vi "Temp Tester for CT.vi"() -> ()   [LabVIEW 2016]
uses:
  type defs/ERD Read List All.ctl
  Q:/Common/DLLs/GEA3/GeaCommunication.dll
  Common/DLLs/GEA3/GeaCommunication.dll
  Common/LabVIEW GEA2 Toolkit/LabVIEW_GEA2_Toolkit.lvlibp/type defs/ERD Read Data Out.ctl
  Common/LabVIEW GEA2 Toolkit/LabVIEW_GEA2_Toolkit.lvlibp/type defs/Source_Destination.ctl
  <vilib>/DAQmx/write.llb/DAQmx Write (Analog 1D DBL NChan 1Samp).vi
  <vilib>/DAQmx/create/channels.llb/DAQmx Create Channel (AO-Voltage-Basic).vi
  <vilib>/DAQmx/miscellaneous.llb/DAQmx Fill In Error Info.vi
  <vilib>/Utility/file.llb/Write Delimited Spreadsheet (DBL).vi
  Common/LabVIEW GEA2 Toolkit/LabVIEW_GEA2_Toolkit.lvlibp
panel:
  out "Array 2":dbl[](array[numeric])
  out "Array":string[](array[string])
  out "ERD Output":T1 {"ERD Number" format="%.0x"}
  in  "Varry Inlet":bool
  in  "Vary Outlet?":bool
  in  "GEA2 Reference In":refnum<k24>
  out "GEA2 Reference Out":refnum<k24>
  out "Error Out":errorcluster
  in  "Delay":u32=2000
  out "error out":errorcluster
  in  "File Path Control":path
  in  "Filtered Moisture":dbl
  in  "ERD Read List ALL":T2=[{"Boolean"=TRUE, "ERD Number"=62475, "ERD Name"="Machine State", "Data Type"=enum."uint8_t"}, {"Boolean"=TRUE, "ERD Number"=62465, "ERD Name"="Relay Status", "Data Type"=enum."string"}, {"Boolean"=TRUE, "ERD Number"=62467, "ERD Name"="Door Switch State", "Data Type"=enum."string"}, {"Boolean"=TRUE, "ERD Number"=62468, "ERD Name"="Door Latch State", "Data Type"=enum."string"}, {"Boolean"=TRUE, "ERD Number"=62469, "ERD Name"="Inlet Thermistor", "Data Type"=enum."int16_t"}, {"Boolean"=TRUE, "ERD Number"=62470, "ERD Name"="Outlet Thermistor", "Data Type"=enum."int16_t"}, {"Boolean"=TRUE, "ERD Number"=62471, "ERD Name"="Filtered Moisture", "Data Type"=enum."int16_t"}, {"Boolean"=TRUE, "ERD Number"=62476, "ERD Name"="Control Lock State", "Data Type"=enum."string"}, {"Boolean"=TRUE, "ERD Number"=62491, "ERD Name"="Signal Volume", "Data Type"=enum."string"}, {"Boolean"=TRUE, "ERD Number"=62478, "ERD Name"="Drum Light", "Data Type"=enum."string"}, {"Boolean"=TRUE, "ERD Number"=62486, "ERD Name"="Delay Time", "Data Type"=enum."string"}, {"Boolean"=TRUE, "ERD Number"=62507, "ERD Name"="Ext. Tumble", "Data Type"=enum."string"}, {"Boolean"=TRUE, "ERD Number"=62487, "ERD Name"="Cycle Time", "Data Type"=enum."uint32_t"}, {"Boolean"=TRUE, "ERD Number"=62488, "ERD Name"="Sub-Cycle", "Data Type"=enum."uint8_t"}, {"Boolean"=TRUE, "ERD Number"=62497, "ERD Name"="Temp Level", "Data Type"=enum."string"}, {"Boolean"=TRUE, "ERD Number"=62499, "ERD Name"="Dryness Level", "Data Type"=enum."string"}, {"Boolean"=TRUE, "ERD Number"=62501, "ERD Name"="eDry", "Data Type"=enum."string"}, {"Boolean"=TRUE, "ERD Number"=62505, "ERD Name"="Time Level", "Data Type"=enum."string"}, {"Boolean"=TRUE, "ERD Number"=62509, "ERD Name"="Damp Alert", "Data Type"=enum."string"}, {"Boolean"=TRUE, "ERD Number"=62511, "ERD Name"="Detangle", "Data Type"=enum."string"}, {"Boolean"=TRUE, "ERD Number"=62520, "ERD Name"="MyCycle", "Data Type"=enum."string"}, {"Boolean"=TRUE, "ERD Number"=62721, "ERD Name"="Cycle Engine State", "Data Type"=enum."string"}, {"Boolean"=TRUE, "ERD Number"=62724, "ERD Name"="Cycle Selected", "Data Type"=enum."string"}] {"ERD Number" format="%.0x"}
  in  "Inlet Temp Voltage":dbl
  in  "Outlet Temp Voltage":dbl
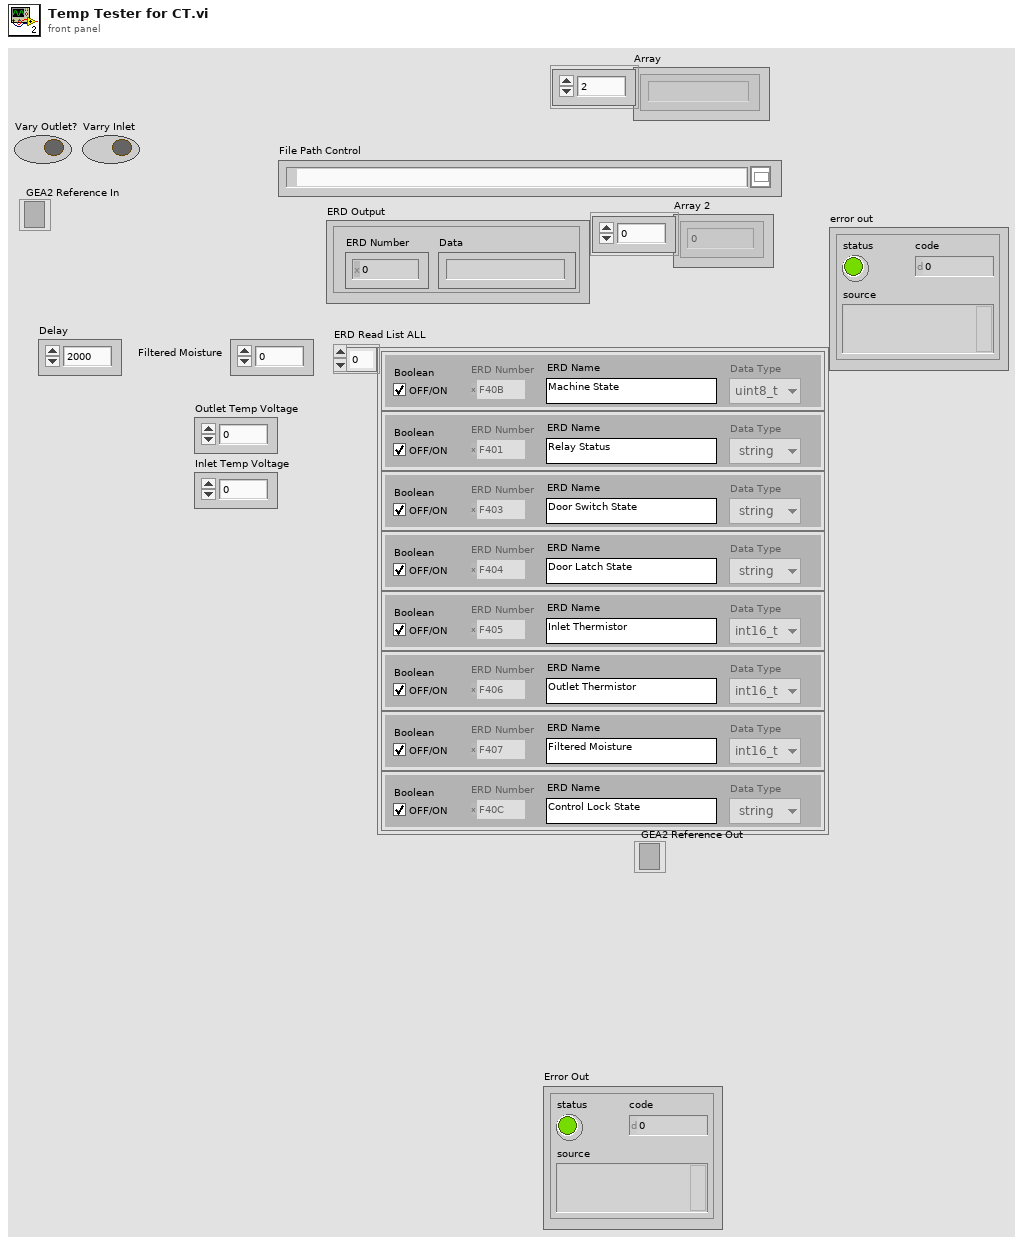
[diagram p1: front panel]
types:
  T1 = typedef "LabVIEW_GEA2_Toolkit.lvlibp/ERD Read Data Out.ctl" = cluster{"ERD Number":u16, "Data":string}
  T2 = typedef "ERD Read List All.ctl" = cluster{"Boolean":bool, "ERD Number":u16, "ERD Name":string, "Data Type":enum16{"string", "boolean", "uint8_t", "uint16_t", "uint32_t", "uint64_t", "int8_t", "int16_t", "int32_t", "int64_t"}}[]
  T3 = enum16{"open", "replace", "create", "open or create", "replace or create", "replace or create with confirmation"}
  T4 = enum16{"Init DAQ", "Build ERD List", "Set Voltage", "Read ERDs ", "Log Data", "Shut Down"}
  T5 = typedef "LabVIEW_GEA2_Toolkit.lvlibp/Source_Destination.ctl" = cluster{"Source":u8, "Destination":u8}
  T6 = typedef "LabVIEW_GEA2_Toolkit.lvlibp/ERD Read Data In.ctl" = cluster{"ERD Number":u16, "Data Type":T7}
  T7 = typedef "LabVIEW_GEA2_Toolkit.lvlibp/Data Type.ctl" = enum16{"string", "boolean", "uint8_t", "uint16_t", "uint32_t", "uint64_t", "int8_t", "int16_t", "int32_t", "int64_t"}
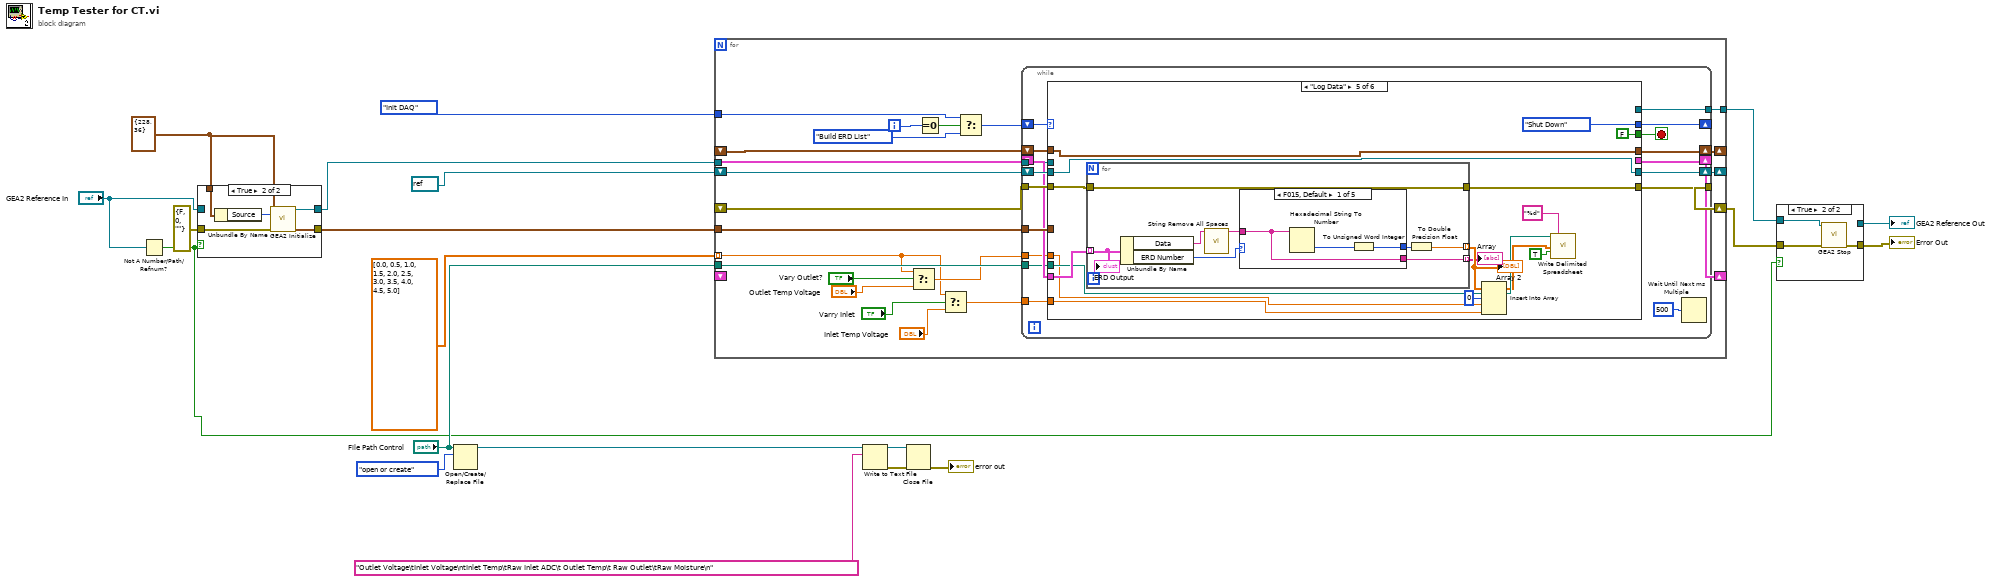
[diagram p0: block diagram]
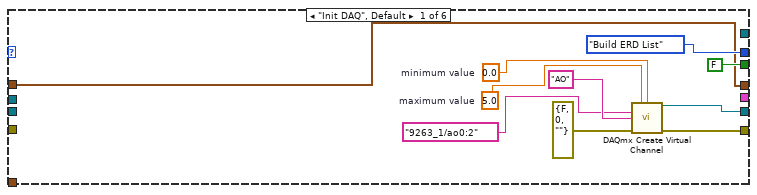
[diagram p4: hidden frame]
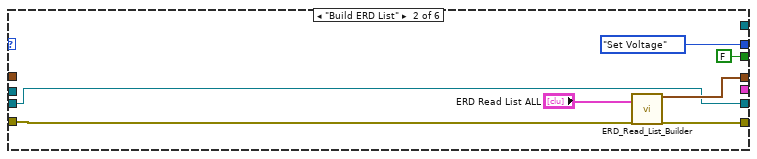
[diagram p5: hidden frame]
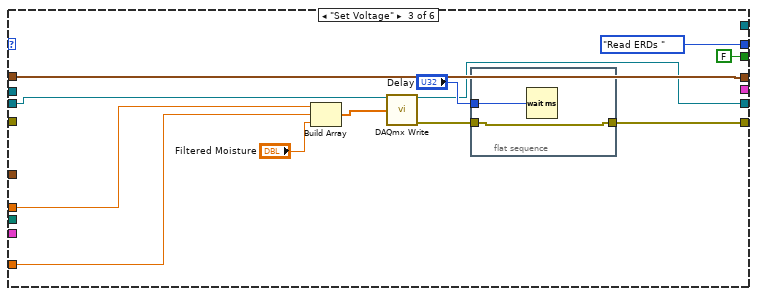
[diagram p6: hidden frame]
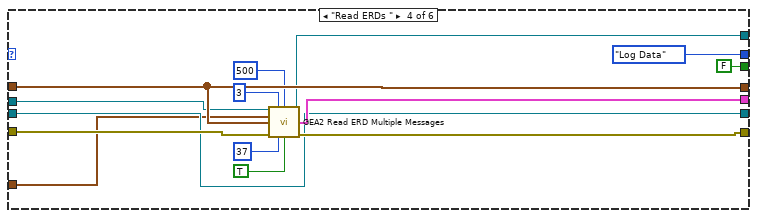
[diagram p7: hidden frame]
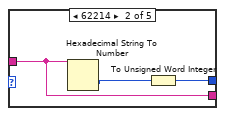
[diagram p8: hidden frame]
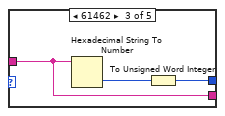
[diagram p9: hidden frame]
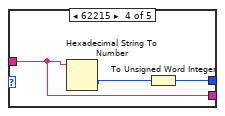
[diagram p10: hidden frame]
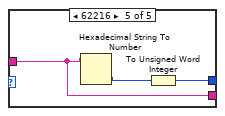
[diagram p11: hidden frame]
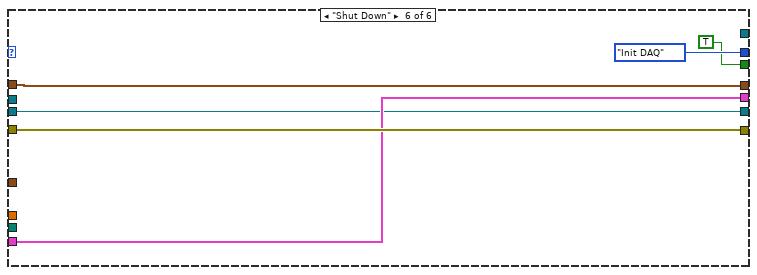
[diagram p12: hidden frame]
diagram:
  w8 = T5 {"Source"=228, "Destination"=36} ("GEA Inputs")
  n1 = Not A Number/Path/Refnum?(number/path/refnum="GEA2 Reference In") -> (NaN/Path/Refnum?=w4:bool)
  n2 = case shown="True" w4 {
    tunnel: errorcluster {"status"=FALSE, "code"=0, "source"=""} ("Error In") -> [w20 w26]
    tunnel: [w20 w25] -> _
    tunnel: "GEA2 Reference In" -> [w21 _]
    tunnel: [w21 w24] -> w9
    tunnel: w8 -> [_ w22]
    frame False {
    }
    frame True {
      n3 = Unbundle By Name(w22) -> ("Source"=w23:u8)
      n4 = call "GEA2 Initialize.vi"("Source Address"=w23, "error in"=w26) -> ("GEA2 Reference Out"=w24:refnum<k24>, "error out"=w25:errorcluster)  [unwired: 11 in, 1 out]
    }
  }
  n5 = Open/Create/Replace File(file path (use dialog)="File Path Control", operation (0:open)=T3."open or create") -> (refnum out=w15:refnum<file>)  [unwired: 4 in, 2 out]
  n6 = for {
    tunnel: w8 -> [w37]
    shift-right: [w38] -> _
    shift-left: refnum<k21> refnum ("task out") -> [w50]
    shift-right: [w49] -> w5
    shift-left: _ -> [w36]
    shift-right: [w48] -> _
    shift-left: _ -> [w47]
    shift-right: [w46] -> _
    shift-left: _ -> [w45]
    tunnel: dbl[] [0.0, 0.5, 1.0, 1.5, 2.0, 2.5, 3.0, 3.5, 4.0, 4.5, 5.0] -> [w32] mode=indexing
    tunnel: "File Path Control" -> [w44]
    tunnel: T4."Init DAQ" -> [w40]
    tunnel: w9 -> [w35]
    tunnel: [w34] -> w2
    i -> [w43]
    n7 = Select(t=w32, s="Vary Outlet?", f="Outlet Temp Voltage") -> (s? t:f=w33:dbl)
    n8 = Equal To 0?(x=w43) -> (x = 0?=w42:bool)
    n9 = Select(t=w32, s="Varry Inlet", f="Inlet Temp Voltage") -> (s? t:f=w31:dbl)
    n10 = Select(t=w40, s=w42, f=T4."Build ERD List") -> (s? t:f=w39:T4)
    n11 = while {
      tunnel: w37 -> [w65]
      tunnel: [w64] -> w49
      tunnel: w36 -> [w63]
      tunnel: w33 -> [w58]
      shift-right: [w67] -> _
      shift-left: w39 -> [w68]
      tunnel: w44 -> [w56]
      shift-right: [w55] -> w38
      shift-left: w50 -> [w66]
      tunnel: w35 -> [w53]
      shift-right: [w60] -> w46
      shift-left: w45 -> [w59]
      tunnel: [w52] -> w34
      shift-right: [w62] -> w48
      shift-left: w47 -> [w61]
      tunnel: w31 -> [w51]
      stop <- w57 stop-if-true
      n12 = case shown="\"Log Data\"" w68 {
        tunnel: [w75 w84 w91 w113 w124 w158] -> w64
        tunnel: [T4."Build ERD List" T4."Set Voltage" T4."Read ERDs " T4."Log Data" T4."Shut Down" T4."Init DAQ"] -> w67
        tunnel: [w72 w81 w89 w108 w129 w156] -> w55
        tunnel: w66 -> [_ w81 w88 w108 w129 w156]
        tunnel: w65 -> [_ _ _ w103 _ _]
        tunnel: w63 -> [_ w80 _ w112 w125 w158]
        tunnel: [w69 w82 w94 w109 w128 w155] -> w62
        tunnel: w61 -> [w69 _ w94 w109 w128 w155]
        tunnel: [_ _ _ w111 _ w157] -> w60
        tunnel: w59 -> [_ _ _ _ w126 w157]
        tunnel: w58 -> [_ _ w93 _ w118 _]
        tunnel: [FALSE FALSE FALSE FALSE FALSE TRUE] -> w57
        tunnel: w56 -> [_ _ _ _ w122 _]
        tunnel: w53 -> [_ _ _ w101 _ _]
        tunnel: [_ _ _ w100 _ _] -> w52
        tunnel: w51 -> [_ _ w86 _ w119 _]
        frame "Init DAQ", Default {
          w77 = 0.0  # minimum value
          w76 = 5.0  # maximum value
          n13 = call-poly <vilib>:"DAQmx Create Virtual Channel.vi"("maximum value"=w76, "minimum value"=w77, "physical channels"=tag "9263_1/ao0:2", "name to assign"="AO", "error in"=errorcluster {"status"=FALSE, "code"=0, "source"=""}) -> ("task out"=w72:refnum<k21>, "error out"=w75:errorcluster)  [unwired: 9 in]
        }
        frame "Build ERD List" {
          n14 = call "ERD_Read_List_Builder.vi"("ERD Read List"="ERD Read List ALL", "Error In"=w80) -> ("Read ERD List"=w82:T6[], "Error Out"=w84:errorcluster)  [unwired: 15 in, 1 out]
        }
        frame "Set Voltage" {
          n15 = Build Array(w93, w86, "Filtered Moisture") -> (w97:dbl[])
          n16 = call-poly <vilib>:"DAQmx Write.vi"("task/channels in"=w88, "data"=w97) -> ("task out"=w89:refnum<k21>, "error out"=w92:errorcluster)  [unwired: 11 in, 1 out]
          n17 = flat-sequence {
            tunnel: w92 -> [w99]
            tunnel: [w99] -> w91
            tunnel: "Delay" -> [w98]
            frame #0 {
              n18 = Wait (ms)(milliseconds to wait=w98) -> ()  [unwired: 1 out]
            }
          }
        }
        frame "Read ERDs " {
          n19 = call "GEA2 Read ERD Multiple Messages.vi"("GEA2 Reference In"=w101, "Retry Count"=3, "Read Timeout (ms)"=u32 500, "GEA Inputs"=w103, "Read ERD List"=w109, "Error In"=w112, "#ERDs per message"=37, "Verify ERD Response?"=TRUE) -> ("GEA2 Reference Out"=w100:refnum<k24>, "ERD Data Out"=w111:T1[], "Error Out"=w113:errorcluster)  [unwired: 4 in, 1 out]
        }
        frame "Log Data" {
          n20 = for {
            tunnel: w126 -> [w137] mode=indexing
            tunnel: w125 -> [w135]
            tunnel: [w135] -> w124
            tunnel: [w131] -> w120 mode=indexing
            tunnel: [w130] -> w114 mode=indexing
            n21 = Unbundle By Name(w137) -> ("Data"=w134:string, "ERD Number"=w136:u16)
            n22 = call "String Remove All Spaces.vi"("Input String"=w134) -> ("Spaces Removed"=w133:string)  [unwired: 13 in, 1 out]
            n23 = case shown="F015, Default" w136 {
              tunnel: w133 -> [w138 w142 w144 w148 w151]
              tunnel: [w139 w143 w145 w149 w152] -> w132
              tunnel: [w138 w142 w144 w148 w151] -> w130
              frame 61461, Default {
                n24 = Hexadecimal String To Number(string=w138) -> (number=w140:u32)  [unwired: 2 in, 1 out]
                n25 = To Unsigned Word Integer(number=w140) -> (unsigned 16bit integer=w139:u16)
              }
              frame 62214 {
                n26 = Hexadecimal String To Number(string=w142) -> (number=w141:u32)  [unwired: 2 in, 1 out]
                n27 = To Unsigned Word Integer(number=w141) -> (unsigned 16bit integer=w143:u16)
              }
              frame 61462 {
                n28 = Hexadecimal String To Number(string=w144) -> (number=w146:u32)  [unwired: 2 in, 1 out]
                n29 = To Unsigned Word Integer(number=w146) -> (unsigned 16bit integer=w145:u16)
              }
              frame 62215 {
                n30 = Hexadecimal String To Number(string=w148) -> (number=w147:u32)  [unwired: 2 in, 1 out]
                n31 = To Unsigned Word Integer(number=w147) -> (unsigned 16bit integer=w149:u16)
              }
              frame 62216 {
                n32 = Hexadecimal String To Number(string=w151) -> (number=w150:u32)  [unwired: 2 in, 1 out]
                n33 = To Unsigned Word Integer(number=w150) -> (unsigned 16bit integer=w152:u16)
              }
            }
            n34 = To Double Precision Float(number=w132) -> (double precision float=w131:dbl)
            "ERD Output" <- w137
          }
          "Array" <- w114
          "Array 2" <- w120
          n35 = Insert Into Array(array=w120, index=0, new element #1=w118, new element #2=w119) -> (w117:dbl[])
          n36 = call-poly <vilib>:"Write Delimited Spreadsheet.vi"("file path (dialog if empty)"=w122, "format (%.3f)"="%d" ("format (%d)"), "1D data"=w117, "append to file? (new file:F)"=TRUE) -> ()  [unwired: 10 in, 2 out]
        }
        frame "Shut Down" {
        }
      }
      n37 = Wait Until Next ms Multiple(millisecond multiple=u32 500) -> ()  [unwired: 1 out]
    }
  }
  n38 = Write to Text File(file (use dialog)=w15, text="Outlet Voltage\tInlet Voltage\ntInlet Temp\tRaw Inlet ADC\t Outlet Temp\t Raw Outlet\tRaw Moisture\n") -> (refnum out=w12:refnum<file>, error out=w13:errorcluster)  [unwired: 2 in, 1 out]
  n39 = Close File(refnum=w12, error in=w13) -> (error out=→"error out":errorcluster)  [unwired: 1 out]
  n40 = case shown="True" w4 {
    tunnel: [w160 w163] -> w7
    tunnel: w2 -> [w159 w161]
    tunnel: w5 -> [w160 w162]
    tunnel: [w159 _] -> w1
    frame False {
    }
    frame True {
      n41 = call "GEA2 Stop.vi"("GEA2 Reference In"=w161, "Error In"=w162) -> ("Error Out"=w163:errorcluster)  [unwired: 13 in]
    }
  }
  "Error Out" <- w7
  "GEA2 Reference Out" <- w1
